vi "add dual gating initalize(SubVI).vi"(9 "字符串":string, 10 "model":string="Delta") -> (0 "连接的字符串":string, 3 "ok or cancel":bool=TRUE)   [LabVIEW 2019, in "Add Seq.lvlib"]
uses:
  Add Seq.lvlib
panel:
  in  "Current Limit B (0.1 A) 2":dbl=0.1
  in  "Current Limit A (0.1 A)":dbl=0.1
  out "错误输出":errorcluster
  in  "load":bool
  in  "cancel":bool
  in  "ok":bool
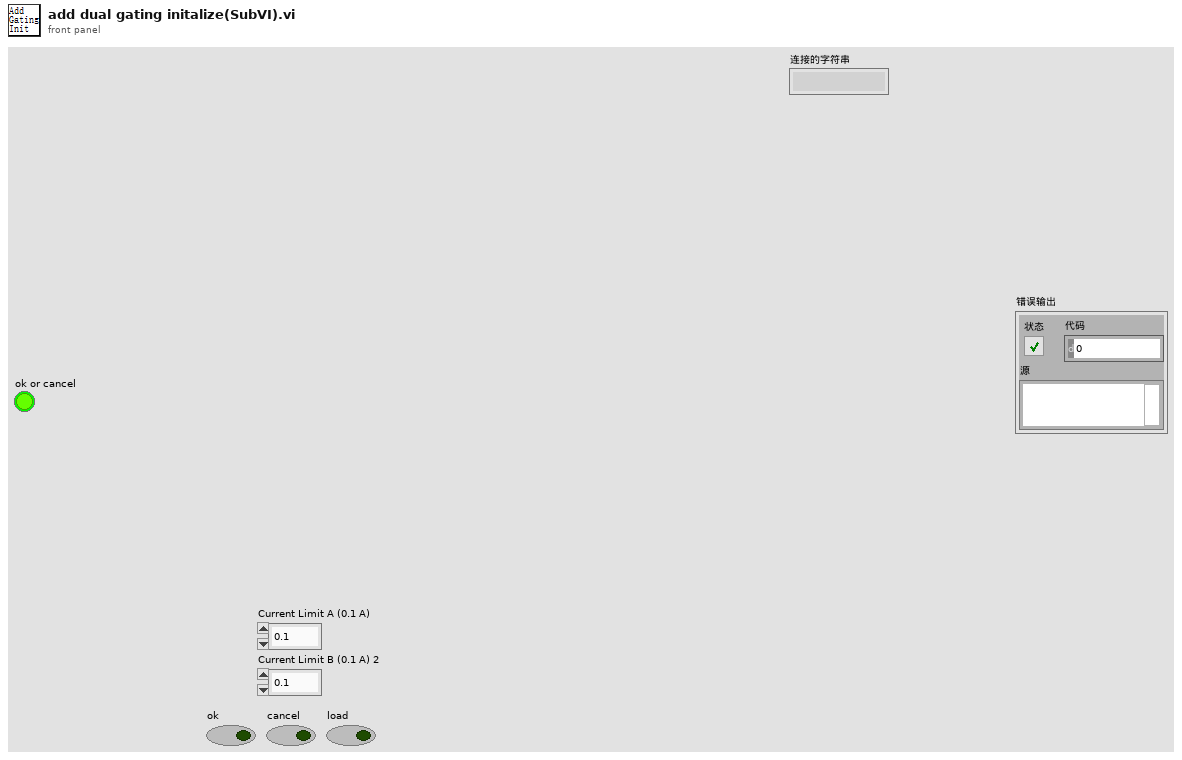
[diagram p1: front panel]
types:
  T1 = enum16{"open", "replace", "create", "open or create", "replace or create"}
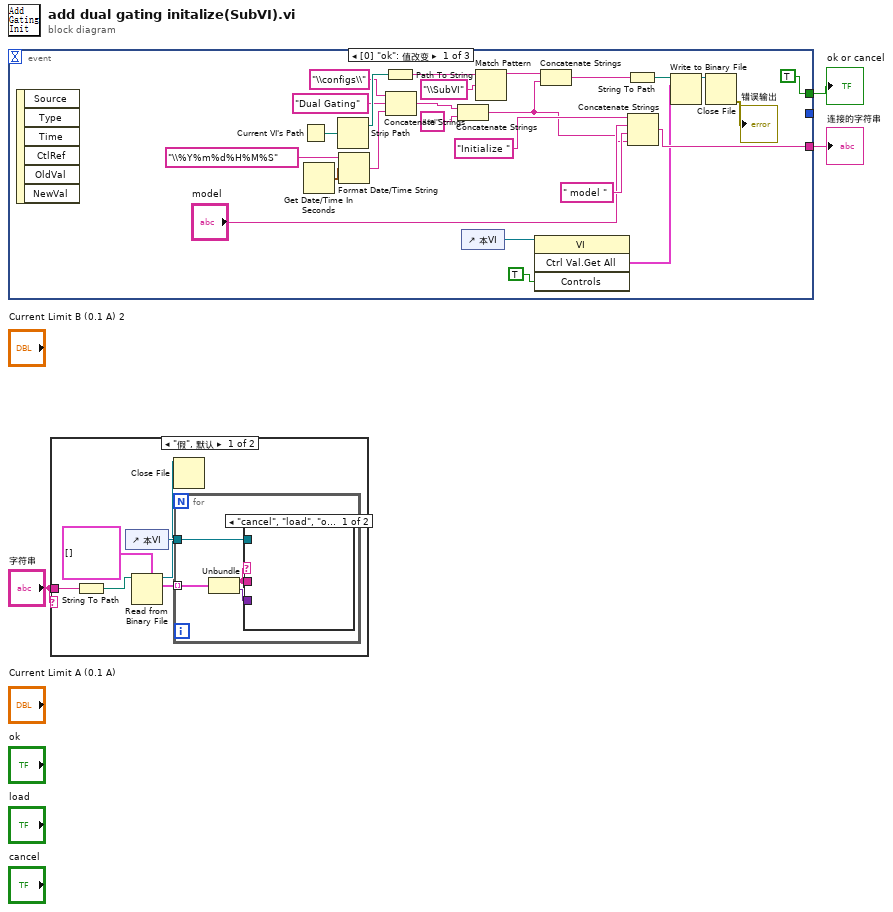
[diagram p0: block diagram]
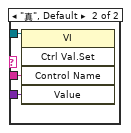
[diagram p2: hidden frame]
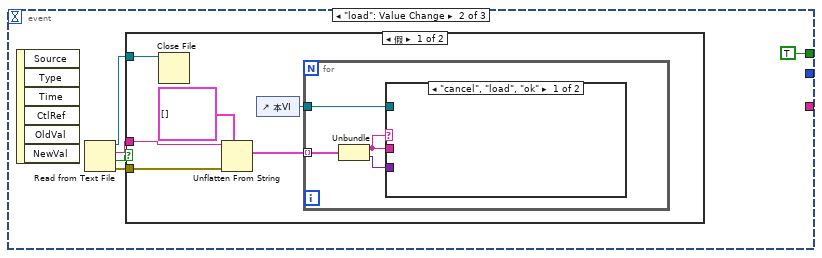
[diagram p4: hidden frame]
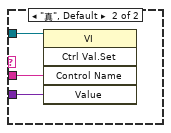
[diagram p5: hidden frame]
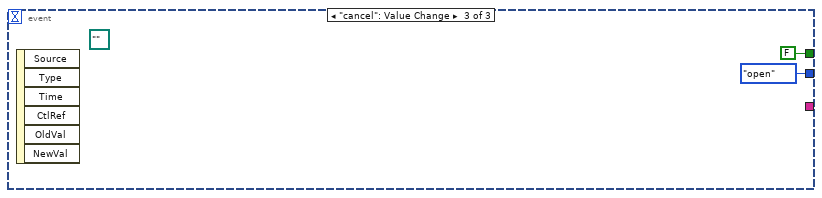
[diagram p7: hidden frame]
diagram:
  n1 = event shown="[0] \"ok\": 值改变" {
    selector: _ -> [_ _ _]
    dyn-events: _ -> [_ _ _]
    timeout: _ -> [_ _ _]
    tunnel: [_ _ T1."open" ("operation(0:open)")] -> _
    tunnel: [TRUE TRUE FALSE] -> w3
    tunnel: [w20 _ _] -> w1
    event "ok": Value Change {
      n2 = event-data() -> ()  [unwired: 1 in, 6 out]
      n3 = Current VI's Path() -> (path=w11:path)
      n4 = Get Date/Time In Seconds() -> (seconds since 1Jan1904=w13:timestamp)
      n5 = Strip Path(path=w11) -> (stripped path=w16:path)  [unwired: 1 out]
      n6 = Format Date/Time String(time format string (%c)="\\%Y%m%d%H%M%S", seconds (now)=w13) -> (date/time string=w12:string)  [unwired: 1 in]
      n7 = Path To String(path=w16) -> (string=w10:string)
      n8 = Concatenate Strings("\\configs\\" ("字符串"), "Dual Gating" ("字符串"), w12) -> (w8:string)
      n9 = Concatenate Strings(w8, ".ini" ("字符串")) -> (w5:string)
      n10 = control-ref of="本VI"() -> (w27:refnum<vi>)
      n11 = Match Pattern(string=w10, regular expression="\\SubVI" ("正则表达式")) -> (before substring=w6:string)  [unwired: 1 in, 3 out]
      n12 = invoke class="VI" method="Ctrl Val.Get All"(reference=w27, "Controls"=TRUE ("控件")) -> ("Get All Control Values Variant"=w18:cluster{"Name":string, "Variant Data":variant}[])  [unwired: 2 in, 3 out]
      n13 = Concatenate Strings(w6, w5) -> (w4:string)
      n14 = String To Path(string=w4) -> (path=w19:path)
      n15 = Concatenate Strings("Initialize " ("字符串"), "model", " model " ("字符串"), w5) -> (w20:string)
      n16 = Write to Binary File(file (use dialog)=w19, data=w18) -> (refnum out=w17:refnum<file>)  [unwired: 4 in, 2 out]
      n17 = Close File(refnum=w17) -> (error out=→"错误输出":errorcluster)  [unwired: 1 in, 1 out]
    }
    event "load": Value Change {
      n18 = event-data() -> ()  [unwired: 1 in, 6 out]
      n19 = Read from Text File() -> (refnum out=w32:refnum<file>, text=w30:string, cancelled=w29:bool, error out=w31:errorcluster)  [unwired: 4 in]
      n20 = case shown="假" w29 {
        tunnel: w32 -> [w39 _]
        tunnel: w31 -> [w37 _]
        tunnel: w30 -> [w36 _]
        frame False {
          n21 = Close File(refnum=w39) -> ()  [unwired: 1 in, 2 out]
          n22 = Unflatten From String(type=cluster{"Name":string, "Variant Data":variant}[] [] ("控件值:获取全部"), binary string=w36, error in (no error)=w37) -> (value=w35:cluster{"Name":string, "Variant Data":variant}[])  [unwired: 2 in, 2 out]
          n23 = control-ref of="本VI"() -> (w34:refnum<vi>)
          n24 = for {
            tunnel: w35 -> [w43] mode=indexing
            tunnel: w34 -> [w42]
            n25 = Unbundle(w43) -> ("Name"=w40:string, "Variant Data"=w41:variant)
            n26 = case shown="\"cancel\", \"load\", \"ok\"" w40 {
              tunnel: w42 -> [_ w46]
              tunnel: w40 -> [_ w45]
              tunnel: w41 -> [_ w44]
              frame "cancel", "load", "ok" {
              }
              frame "真", Default {
                n27 = invoke class="VI" method="Ctrl Val.Set"(reference=w46, "Control Name"=w45, "Value"=w44) -> ()  [unwired: 2 in, 5 out]
              }
            }
          }
        }
        frame True {
        }
      }
    }
    event "cancel": Value Change {
      (unwired) path "" ("path")
      n28 = event-data() -> ()  [unwired: 1 in, 6 out]
    }
  }
  "ok or cancel" <- w3
  "连接的字符串" <- w1
  n29 = case shown="\"假\", 默认" "字符串" {
    tunnel: "字符串" -> [w54 _]
    frame "假", Default {
      n30 = String To Path(string=w54) -> (path=w52:path)
      n31 = control-ref of="本VI"() -> (w53:refnum<vi>)
      n32 = Read from Binary File(5:cluster{"Name":string, "Variant Data":variant}[] [] ("控件值:获取全部"), 11:w52) -> (2:w50:cluster{"Name":string, "Variant Data":variant}[], 3:w49:refnum<file>)  [unwired: 4 in, 2 out]
      n33 = Close File(refnum=w49) -> ()  [unwired: 1 in, 2 out]
      n34 = for {
        tunnel: w50 -> [w58] mode=indexing
        tunnel: w53 -> [w57]
        n35 = Unbundle(w58) -> ("Name"=w55:string, "Variant Data"=w56:variant)
        n36 = case shown="\"cancel\", \"load\", \"ok\"" w55 {
          tunnel: w57 -> [_ w61]
          tunnel: w55 -> [_ w60]
          tunnel: w56 -> [_ w59]
          frame "cancel", "load", "ok" {
          }
          frame "真", Default {
            n37 = invoke class="VI" method="Ctrl Val.Set"(reference=w61, "Control Name"=w60, "Value"=w59) -> ()  [unwired: 2 in, 5 out]
          }
        }
      }
    }
    frame "" {
    }
  }
